vi "Set Registry Data.vi"(8 "error in (no error)":errorcluster, 10 "Registry Data":variant, 11 "Registry in":refnum<class "Registry.lvclass">) -> (0 "error out":errorcluster, 3 "Registry out":refnum<class "Registry.lvclass">)   [LabVIEW 2020, in "BCI-1553 API.lvlib" / "Registry.lvlib" / "Registry.lvclass"]
doc: "Directly set the variant used by the Registry for Key/Value storage."
uses:
  Registry.lvclass
  Registry.lvclass/Registry.ctl
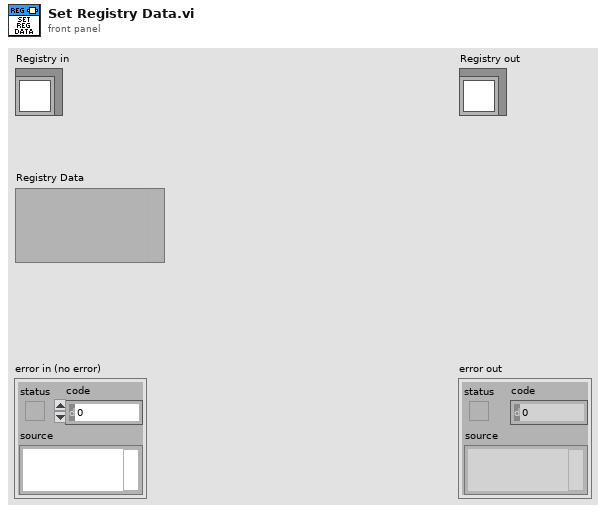
[diagram p1: front panel]
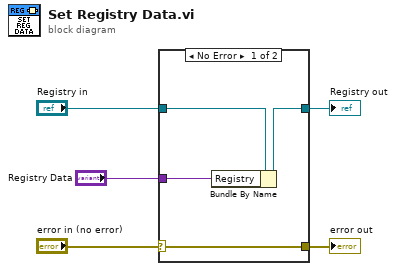
[diagram p0: block diagram]
diagram:
  n1 = case shown="No Error" "error in (no error)" {
    selector: "error in (no error)" -> [w9 w11]
    tunnel: [w9 w11] -> w4
    tunnel: [w6 w10] -> w2
    tunnel: "Registry in" -> [w7 w10]
    tunnel: "Registry Data" -> [w8 _]
    frame No Error {
      n2 = Bundle By Name(cluster=w7, "Registry"=w8) -> (w6:refnum<class "Registry.lvclass">)
    }
    frame Error {
    }
  }
  "error out" <- w4
  "Registry out" <- w2
